vi "test.vi"   [LabVIEW 2019, in "SLMP.lvlib" / "SLMP.lvclass"]
uses:
  SLMP.lvclass
  Device/Device.lvclass
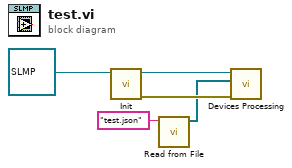
[diagram p0: block diagram]
diagram:
  n1 = call "Init.vi"("SLMP in"=refnum<class "SLMP.lvclass"> refnum ("SLMP.lvlib:SLMP.lvclass")) -> ("error out"=w3:errorcluster, "SLMP out"=w4:refnum<class "SLMP.lvclass">)  [unwired: 9 in]
  n2 = call "Read from File.vi"("Config name"="test.json") -> ("Devices"=w2:refnum<class "Device.lvclass">[])  [unwired: 10 in]
  n3 = call "Devices Processing.vi"("error in (no error)"=w3, "Devices"=w2, "SLMP in"=w4) -> ()  [unwired: 7 in, 2 out]
